vi "Selector.vi"(7 "Name":string="Selector", 11 "Nodes":refnum<class "abs_Node.lvclass">[](array[class])) -> (3 "Node":refnum<class "abs_Node.lvclass">)   [LabVIEW 2021, in "BT.lvlib"]
uses:
  BT.lvlib
  abs_Node/abs_Node.lvclass
  Selector/Selector.lvclass
  C:/Users/Tim/Documents/LabVIEW/2021/Behaviour Tree/abs_Composite/abs_Composite.lvclass
  C:/Users/Tim/Documents/LabVIEW/2021/Behaviour Tree/abs_Node/abs_Node.lvclass
  abs_Composite/abs_Composite.lvclass/abs_Composite.ctl
  abs_Node/abs_Node.lvclass/abs_Node.ctl
  abs_Composite/Properties/Write Nodes.vi
  abs_Node/Properties/Write Name.vi
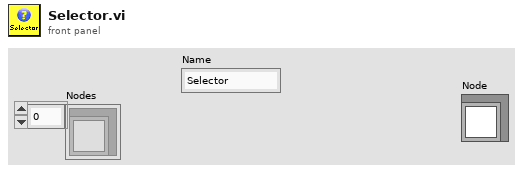
[diagram p1: front panel]
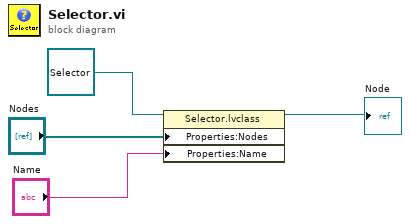
[diagram p0: block diagram]
diagram:
  n1 = property class="Selector.lvclass"(reference=refnum<class "Selector.lvclass"> refnum ("BT.lvlib:Selector.lvclass"), "Properties:Nodes"="Nodes", "Properties:Name"="Name") -> (reference out=→"Node":refnum<class "Selector.lvclass">)  [unwired: 1 in, 1 out]
